vi "Update Tasks.vi"(8 "error in (no error)":errorcluster, 10 "Task List":refnum<class "Task.lvclass">[](array[class]), 11 "BuildServer in":refnum<class "BuildServer.lvclass">) -> (0 "error out":errorcluster, 3 "BuildServer out":refnum<class "BuildServer.lvclass">)   [LabVIEW 2017, in "BuildServer.lvlib" / "BuildServer.lvclass"]
uses:
  BuildServer.lvclass
  <vilib>/ActorFramework/Actor/Actor.lvclass
  BuildServer Messages/Update TaskView Msg/Update TaskView Msg.lvclass
  Volumes/Data/Users/benji667/Git/BuildFarm/src/LabVIEW/vi.lib/BenjaminR/Build Farm/Actors/Framework/Actor wHelper/Actor wHelper.lvclass
  Volumes/Data/Users/benji667/Git/BuildFarm/src/LabVIEW/vi.lib/BenjaminR/Build Farm/Actors/Framework/Actor wLauncher/Actor wLauncher.lvclass
  Volumes/Data/Users/benji667/Git/BuildFarm/src/LabVIEW/vi.lib/BenjaminR/Build Farm/Actors/Framework/Actor wUI/Actor wUI.lvclass
  Applications/National Instruments/LabVIEW 2017 64-bit/vi.lib/ActorFramework/Actor/Actor.lvclass
  Classes/Task Interface/Task/Task.lvclass
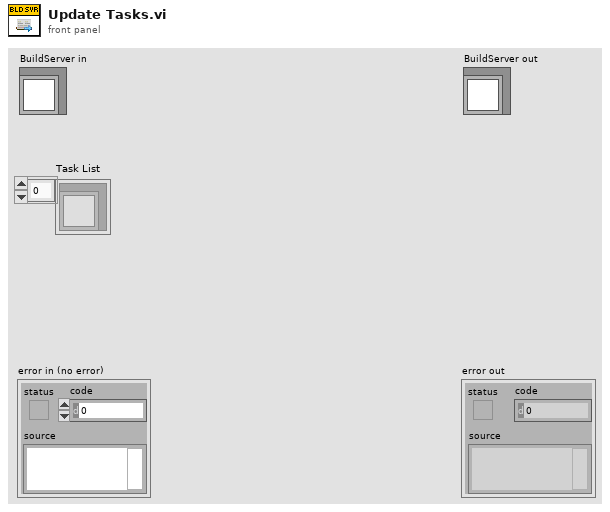
[diagram p1: front panel]
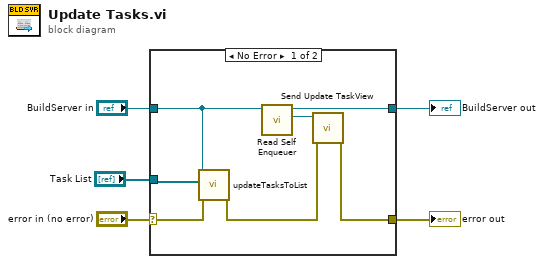
[diagram p0: block diagram]
diagram:
  n1 = case shown="No Error" "error in (no error)" {
    selector: "error in (no error)" -> [w10 w13]
    tunnel: [w6 w13] -> w4
    tunnel: [w8 w12] -> w2
    tunnel: "BuildServer in" -> [w8 w12]
    tunnel: "Task List" -> [w11 _]
    frame No Error {
      n2 = call "updateTasksToList.vi"("error in (no error)"=w10, "Selected Tasks"=w11, "BuildServer in"=w8) -> ("error out"=w7:errorcluster)  [unwired: 8 in]
      n3 = call <vilib>:"Read Self Enqueuer.vi"("Actor"=w8) -> ("Self Enqueuer"=w9:refnum<class "Message Enqueuer.lvclass">)  [unwired: 10 in]
      n4 = call "Send Update TaskView.vi"("error in (no error)"=w7, "Message Enqueuer"=w9) -> ("error out"=w6:errorcluster)  [unwired: 8 in, 1 out]
    }
    frame Error {
    }
  }
  "error out" <- w4
  "BuildServer out" <- w2
